vi "Mixer.Connect Monitor.vi"(7 "source":i32) -> ()   [LabVIEW 2020]
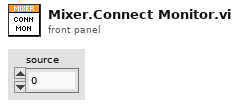
[diagram p1: front panel]
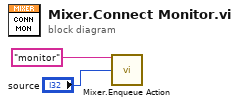
[diagram p0: block diagram]
diagram:
  n1 = call "Mixer.Enqueue Action.vi"("action"="monitor", "data"="source") -> ()  [unwired: 13 in, 1 out]
